vi "Obliczenia enkoderow.vi"(8 "error in (no error)":errorcluster, 10 "Enkoder in":waveform(dbl)[](array[waveform])) -> (0 "error out":errorcluster, 2 "Enkoder out":waveform(dbl)[](array[waveform]))   [LabVIEW 2014]
doc: "Use this template to build a VI to use as a subVI."
uses:
  Kontrolki/GUI/Enkoder Data.ctl
  Kontrolki/FVGs/FVG akcje podstawowa.ctl
panel:
  in  "Akcja":bool
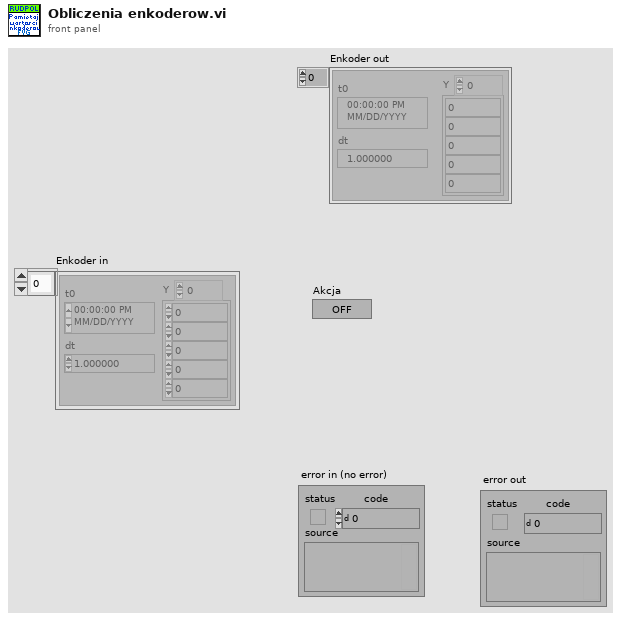
[diagram p1: front panel]
types:
  T1 = typedef "Enkoder Data.ctl" = cluster{"d":dbl, "v":dbl, "a":dbl}
  T2 = typedef "FVG akcje podstawowa.ctl" = enum16{"GET", "SET"}
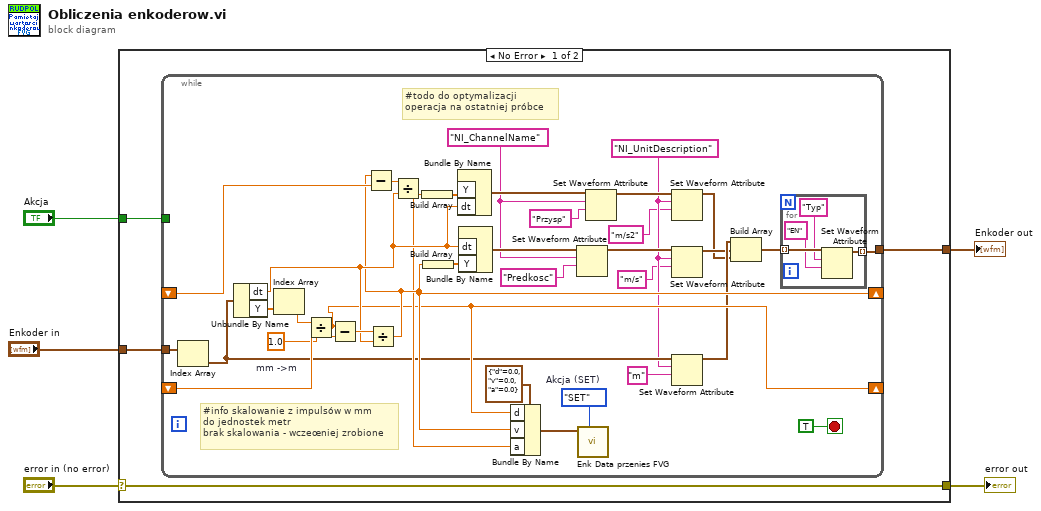
[diagram p0: block diagram]
diagram:
  n1 = case shown="No Error" "error in (no error)" {
    selector: "error in (no error)" -> [w6 w50]
    tunnel: [w6 w50] -> w4
    tunnel: "Enkoder in" -> [w9 w49]
    tunnel: "Akcja" -> [w8 _]
    tunnel: [w7 w49] -> w2
    frame No Error {
      n2 = while {
        tunnel: w9 -> [w43]
        shift-right: [w21] -> _
        shift-left: _ -> [w42]
        tunnel: w8 -> [_]
        shift-right: [w27] -> _
        shift-left: _ -> [w39]
        tunnel: [w23] -> w7
        stop <- TRUE stop-if-true
        w13 = "NI_UnitDescription" ("name")
        w20 = 1.0  # mm ->m
        w25 = FVG_akcje_podstawowa."SET"  # Akcja (SET)
        w36 = "NI_ChannelName" ("name")
        # "#info skalowanie z impulsów w mm\ndo jednostek metr\nbrak skalowania - wczeœniej zrobione"
        # "#todo do optymalizacji\noperacja na ostatniej próbce"
        n3 = Index Array(array=w43) -> (element=w19:waveform(dbl))  [unwired: 1 in]
        n4 = Unbundle By Name(w19) -> ("dt"=w30:dbl, "Y"=w33:dbl[])
        n5 = Index Array(array=w33) -> (element=w22:dbl)  [unwired: 1 in]
        n6 = Divide(x=w22, y=w20) -> (x/y=w21:dbl)
        n7 = Subtract(x=w21, y=w42) -> (x-y=w41:dbl)
        n8 = Divide(x=w41, y=w30) -> (x/y=w27:dbl)
        n9 = Subtract(x=w27, y=w39) -> (x-y=w40:dbl)
        n10 = Divide(x=w40, y=w30) -> (x/y=w26:dbl)
        n11 = Build Array(w26) -> (w31:dbl[])
        n12 = Build Array(w27) -> (w32:dbl[])
        n13 = Bundle By Name("Y"=w31, "dt"=w30) -> (w37:waveform(dbl))  [unwired: 1 in]
        n14 = Bundle By Name("dt"=w30, "Y"=w32) -> (w38:waveform(dbl))  [unwired: 1 in]
        n15 = Bundle By Name(cluster=T1 {"d"=0.0, "v"=0.0, "a"=0.0} ("Enkoder Data in"), "d"=w21, "v"=w27, "a"=w26) -> (w28:T1)
        n16 = Set Waveform Attribute(5:"Predkosc" ("name"), 6:w36, 7:w38) -> (3:w17:waveform(dbl))  [unwired: 1 in, 2 out]
        n17 = call "Enk Data przenies FVG.vi"("Akcja (SET)"=w25, "Enkoder Data in"=w28) -> ()  [unwired: 8 in, 2 out]
        n18 = Set Waveform Attribute(5:"Przysp" ("name"), 6:w36, 7:w37) -> (3:w15:waveform(dbl))  [unwired: 1 in, 2 out]
        n19 = Set Waveform Attribute(5:"m/s2" ("name"), 6:w13, 7:w15) -> (3:w14:waveform(dbl))  [unwired: 1 in, 2 out]
        n20 = Set Waveform Attribute(5:"m/s" ("name"), 6:w13, 7:w17) -> (3:w16:waveform(dbl))  [unwired: 1 in, 2 out]
        n21 = Set Waveform Attribute(5:"m" ("name"), 6:w13, 7:w19) -> (3:w18:waveform(dbl))  [unwired: 1 in, 2 out]
        n22 = Build Array(w18, w16, w14) -> (w24:waveform(dbl)[])
        n23 = for {
          tunnel: w24 -> [w48] mode=indexing
          tunnel: [w47] -> w23 mode=indexing
          n24 = Set Waveform Attribute(5:"EN", 6:"Typ", 7:w48) -> (3:w47:waveform(dbl))  [unwired: 1 in, 2 out]
        }
      }
    }
    frame Error {
    }
  }
  "error out" <- w4
  "Enkoder out" <- w2
